vi "bool to disabled state (sub-vi).vi"(1 "error?":bool) -> (0 "disabled":T1(ring))   [LabVIEW 2021]
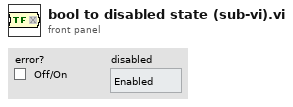
[diagram p1: front panel]
types:
  T1 = enum8{"Enabled", "Disabled", "Disabled and Grayed Out"}
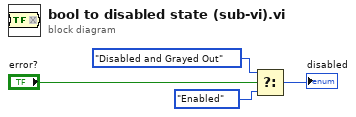
[diagram p0: block diagram]
diagram:
  n1 = Select(t=T1."Disabled and Grayed Out", s="error?", f=T1."Enabled" ("Disabled")) -> (s? t:f=→"disabled":T1)
